vi "calc_lifetime_nomatlab.vi"(1 "unbinned data":u16[][](array[numeric])) -> (0 "lifetimes":sgl[](array[numeric]))   [LabVIEW 2013]
uses:
  <vilib>/Analysis/6fits.llb/Curve Fitting Criteria.ctl
  <vilib>/Analysis/NI_AALPro.lvlib
panel:
  in  "truncate":bool
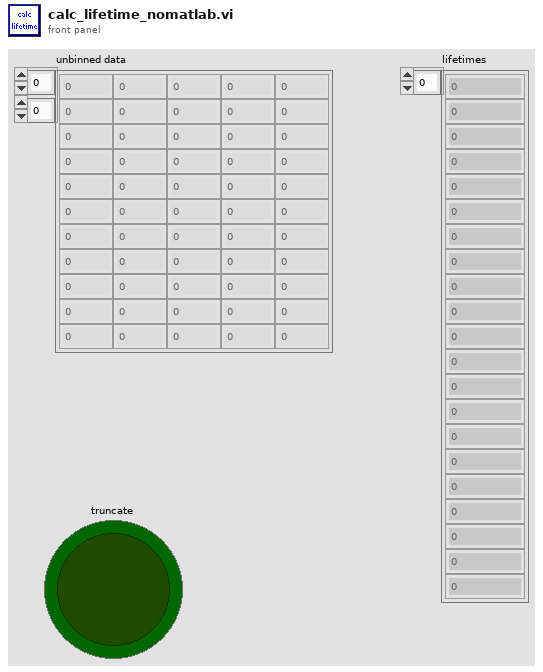
[diagram p1: front panel]
types:
  T1 = typedef "NI_AALPro.lvlib/Curve Fitting Criteria.ctl" = u16
  T2 = cluster{"Z_n":i32[], "devidx":i32, "initialized":bool, "acq time":i32, "Bin size":enum16{"1", "2", "4", "8", "16", "32", "64", "128"}, "# bins":i32, "sync rate":i32, "truncate":bool, "Ch0 Level":i32, "Ch1 Level":i32, "Ch0 ZeroX":i32, "Ch1 ZeroX":i32, "resolution":i32}
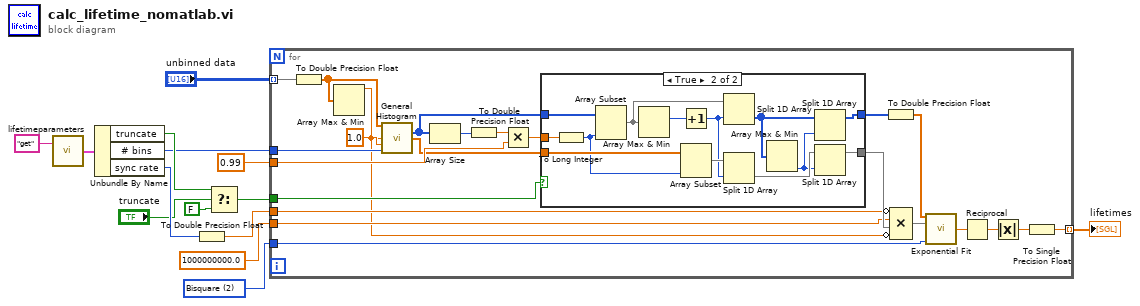
[diagram p0: block diagram]
diagram:
  w4 = T1 2 items=["Least Square", "Least Absolute Residual", "Bisquare"] ("method")
  n1 = call "lifetimeparameters.vi"("command"="get") -> ("Params out"=w13:T2)  [unwired: 1 in]
  n2 = Unbundle By Name(w13) -> ("truncate"=w8:bool, "# bins"=w2:i32, "sync rate"=w10:i32)
  n3 = To Double Precision Float(number=w10) -> (double precision float=w9:dbl)
  n4 = Select(t=w8, s="truncate", f=FALSE) -> (s? t:f=w6:bool)
  n5 = for {
    tunnel: 0.99 ("y") -> [w37]
    tunnel: "unbinned data" -> [w28] mode=indexing
    tunnel: w2 -> [w32]
    tunnel: w6 -> [w27]
    tunnel: 1000000000.0 ("value") -> [w26]
    tunnel: w9 -> [w25]
    tunnel: w4 -> [w18]
    tunnel: [w15] -> w1 mode=indexing
    n6 = To Double Precision Float(number=w28) -> (double precision float=w23:dbl[])
    n7 = Array Max & Min(array=w23) -> (max value=w20:dbl)  [unwired: 3 out]
    n8 = call <vilib>:"General Histogram.vi"("X"=w23, "max"=w20, "min"=1.0, "# bins"=w32) -> ("Histogram"=w31:i32[], "Axis"=w22:dbl[])  [unwired: 7 in, 3 out]
    n9 = Array Size(array=w31) -> (size(s)=w21:i32)
    n10 = To Double Precision Float(number=w21) -> (double precision float=w24:dbl)
    n11 = Multiply(x=w24, y=w37) -> (x*y=w30:dbl)
    n12 = case shown="True" w27 {
      tunnel: [w38 w52] -> w34
      tunnel: [w39 w51] -> w33
      tunnel: w22 -> [w38 w50]
      tunnel: w31 -> [w39 w49]
      tunnel: w30 -> [_ w43]
      frame False {
      }
      frame True {
        n13 = To Long Integer(number=w43) -> (32bit integer=w42:i32)
        n14 = Array Subset(array=w49, length=w42) -> (w48:i32[])  [unwired: 1 in]
        n15 = Array Max & Min(array=w48) -> (max index (indices)=w41:i32)  [unwired: 3 out]
        n16 = Increment(x=w41) -> (x+1=w40:i32)
        n17 = Array Subset(array=w50, length=w42) -> (w44:dbl[])  [unwired: 1 in]
        n18 = Split 1D Array(array=w48, index=w40) -> (second subarray=w47:i32[])  [unwired: 1 out]
        n19 = Split 1D Array(array=w44, index=w40) -> (second subarray=w46:dbl[])  [unwired: 1 out]
        n20 = Array Max & Min(array=w47) -> (min index (indices)=w45:i32)  [unwired: 3 out]
        n21 = Split 1D Array(array=w47, index=w45) -> (first subarray=w51:i32[])  [unwired: 1 out]
        n22 = Split 1D Array(array=w46, index=w45) -> (first subarray=w52:dbl[])  [unwired: 1 out]
      }
    }
    n23 = To Double Precision Float(number=w33) -> (double precision float=w19:dbl[])
    n24 = Compound Arithmetic op=MULTIPLY(invert w25, w26, w34, invert w20) -> (w16:dbl[])
    n25 = call <vilib>:"Exponential Fit.vi"("Y"=w19, "X"=w16, "method"=w18) -> ("damping"=w17:dbl)  [unwired: 7 in, 5 out]
    n26 = Reciprocal(x=w17) -> (1/x=w36:dbl)
    n27 = Absolute Value(x=w36) -> (abs(x)=w35:dbl)
    n28 = To Single Precision Float(number=w35) -> (single precision float=w15:sgl)
  }
  "lifetimes" <- w1
